vi "Delete Scale.vi"(8 "error in (no error)":errorcluster, 10 "Index":i32, 11 "references":T1) -> (0 "error out":errorcluster)   [LabVIEW 2013, in "Scaling editor node.lvclass"]
uses:
  Scaling editor node.lvclass
  <vilib>/NI/DCAF Table API/Table Manager/object ref.ctl
  <vilib>/NI/Tag Bus Data Framework/Configuration Editor/Classes/Engine Parent/Engine Parent Editor Node.lvclass
  <vilib>/NI/Tag Bus Data Framework/Configuration Editor/Classes/Module editor node/module editor node.lvclass
  module/configuration/Scaling configuration.lvclass
  <vilib>/NI/DCAF Table API/Table Manager/Table Manager.lvclass
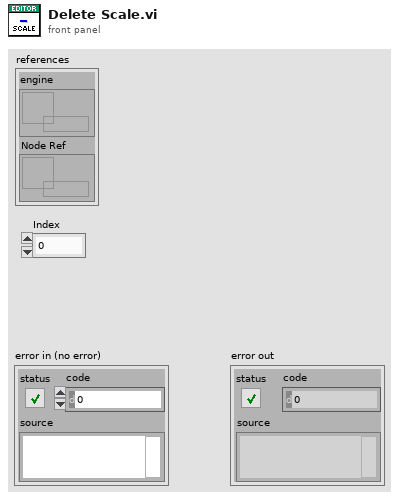
[diagram p1: front panel]
types:
  T1 = typedef "Table Manager.lvlib/Table Manager.lvclass/object ref.ctl" = cluster{"engine":refnum<data-value>, "Node Ref":refnum<data-value>}
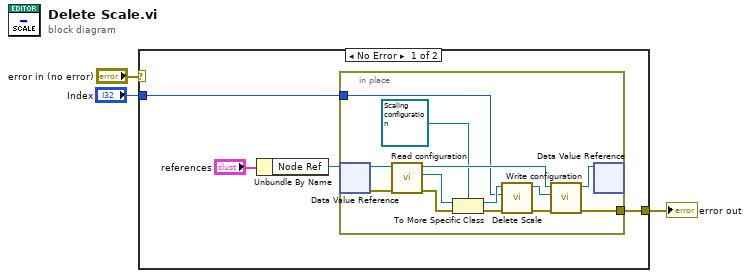
[diagram p0: block diagram]
diagram:
  n1 = case shown="No Error" "error in (no error)" {
    selector: "error in (no error)" -> [_ w21]
    tunnel: [w7 w21] -> w1
    tunnel: "Index" -> [w4 _]
    frame No Error {
      n2 = Unbundle By Name("references") -> ("Node Ref"=w5:refnum<data-value>)
      n3 = in-place {
        in-place-border: [w16] -> w7
        in-place-border: w4 -> [w10]
        n4 = in-place-dvr #1(w5) -> (w19:refnum<class "module editor node.lvclass">, w15:errorcluster)
        n5 = call-dynamic "Read configuration.vi"("error in"=w15, "NISE_CEF_serializable node in"=w19) -> ("error out"=w13:errorcluster, "configuration"=w18:refnum<class "NISE_CEF_serializable configuration.lvclass">, "NISE_CEF_serializable node out"=w20:refnum<class "module editor node.lvclass">)  [unwired: 7 in]
        n6 = To More Specific Class(target class=refnum<class "Scaling configuration.lvclass"> refnum ("Scaling configuration"), reference=w18, error in=w13) -> (specific class reference=w12:refnum<class "Scaling configuration.lvclass">, error out=w11:errorcluster)
        n7 = call-dynamic "Delete Scale.vi"("error in (no error)"=w11, "index"=w10, "Scaling configuration in"=w12) -> ("error out"=w9:errorcluster, "Scaling configuration out"=w8:refnum<class "Scaling configuration.lvclass">)  [unwired: 7 in]
        n8 = call-dynamic "Write configuration.vi"("error in"=w9, "configuration"=w8, "NISE_CEF_serializable node in"=w20) -> ("error out"=w16:errorcluster, "NISE_CEF_serializable node out"=w17:refnum<class "module editor node.lvclass">)  [unwired: 7 in]
        n9 = in-place-dvr #1(w17) -> ()  [unwired: 2 out]
      }
    }
    frame Error {
    }
  }
  "error out" <- w1
